vi "Module (Top Level).vi"(8 "error in":errorcluster) -> (0 "error out":errorcluster)   [LabVIEW 2017, in "myPAM.lvlib"]
uses:
  myPAM.lvlib
  Controls/RT Host - assistance definition.ctl
  Controls/RT Host - assistance options.ctl
  Controls/RT Host - form of control.ctl
  Controls/hCAAR - speed profile.ctl
  Controls/RT Host - assistance settings.ctl
  User Events/TypeDefs/Shutdown UE FGV Command.ctl
  Global TypeDefs/Registered Modules.ctl
  Public TypeDefs/Messages.ctl
  Public TypeDefs/Data for Logging.ctl
  <vilib>/Platform/TimedLoop/XDataNode/timing_clust.ctl
  <vilib>/Platform/TimedLoop/XDataNode/nitl_modes.ctl
  <vilib>/Platform/TimedLoop/XDataNode/wakeup.ctl
  Libraries/Real time filter/TypeDefs/Modes.ctl
  Public TypeDefs/Current Position Data.ctl
  <vilib>/FPGAPlugInAG/myRIO-1900/niLvFpga_Open_myRIO-1900.vi
  <vilib>/Utility/error.llb/Error Cluster From Error Code.vi
  <vilib>/rvi/errors/niLvFpgaAdjustHostInterfaceError.vi
  <vilib>/FPGAPlugInAG/myRIO-1900/niLvFpga_Run_myRIO-1900.vi
  <vilib>/FPGAPlugInAG/myRIO-1900/niLvFpga_Close_myRIO-1900.vi
  <vilib>/rvi/interface/nirviOpenFPGA/nirviOpenFPGA.xnode
  <instrlib>/Devantech SRF02/FPGA Example/Serial/Private/FPGA Reference.ctl
  FPGA Bitfiles/myPAM_FPGATarget_FPGA(TopLevel)_Z9iTYCZN6aI.lvbitx
  FPGA/FPGA (Top Level).vi
  <vilib>/rvi/interface/nirviReadWriteControl/nirviReadWriteControl.xnode
  <vilib>/rvi/interface/nirviMethod/nirviMethod.xnode
  <vilib>/Platform/TimedLoop/XDataNode/XDataNode.xnode
  <vilib>/rvi/interface/nirviCloseFPGA/nirviCloseFPGA.xnode
  Logger/Logger.lvlib
  Error Handler/Error Handler.lvlib
  Game/Game.lvlib
  <vilib>/Platform/TimedLoop/XDataNode/XDNodeRunTimeDep.lvlib
  WinHost/WinHost.lvlib
  Libraries/Real time filter/RealTimeFilter.lvlib
  NiFpgaLv.dll
panel:
  in  "g2":dbl=400.0 format="%#_13g"
  in  "g1":dbl=7100.0 format="%#_13g"
  in  "Parameters":T1={"Spring Stiffness"=9.0, "Deadzone Radius"=0.1, "Damping "=0.09}
  in  "Assistance Definition":T2={"Assistance Options"={"Assist Towards Target?"=TRUE, "Assist Ratchet?"=FALSE, "Form of Control?"=enum."Gen II", "Which Speed Profile?"=enum."Forward Skew"}, "Assistance Settings"={"Max Valley Width (mm)"=30.0, "Valley Width @ Tn (0-0.5)"=0.5, "Valley Width @ Tn-1 (0.5-1)"=0.5, "Valley Depth (0-1)"=1.0, "Stiffness (0-1)"=0.5, "Max Step Increment (mm)"=3.0, "Speed (0-1)"=0.33}}
  in  "Elbow":T7={"Spring Stiffness"=5.0, "Deadzone Radius"=0.01}
  in  "Shoulder":T7={"Spring Stiffness"=4.4, "Deadzone Radius"=0.01}
  out "LINK1_DEMAND":dbl
  out "LINK2_DEMAND":dbl
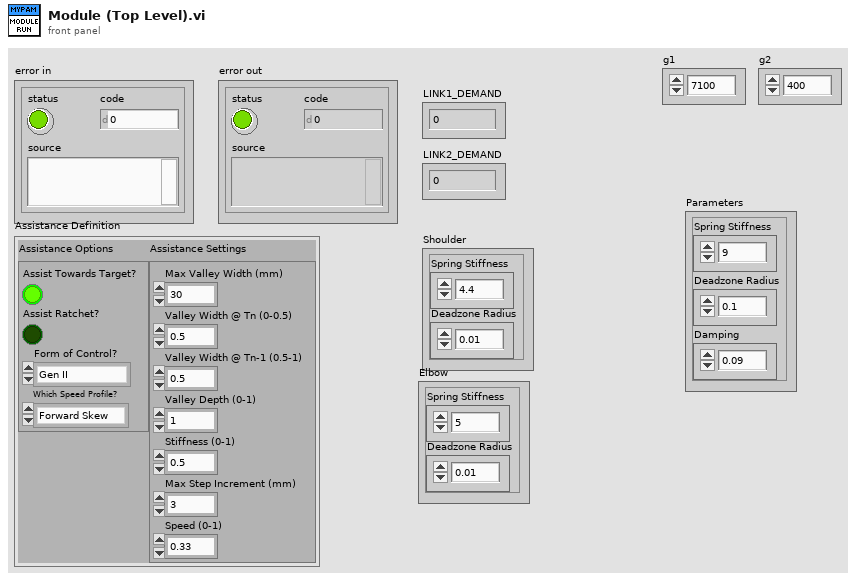
[diagram p1: front panel]
types:
  T1 = cluster{"Spring Stiffness":dbl, "Deadzone Radius":dbl, "Damping ":dbl}
  T2 = typedef "RT Host - assistance definition.ctl" = cluster{"Assistance Options":T3, "Assistance Settings":T6}
  T3 = typedef "RT Host - assistance options.ctl" = cluster{"Assist Towards Target?":bool, "Assist Ratchet?":bool, "Form of Control?":T4, "Which Speed Profile?":T5}
  T4 = typedef "RT Host - form of control.ctl" = enum16{"Baseline", "Gen II", "No Assist"}
  T5 = typedef "hCAAR - speed profile.ctl" = enum16{"Sine", "Sine With Initial Shunt", "Triangle", "Square", "Sawtooth", "Forward Skew", "User Defined"}
  T6 = typedef "RT Host - assistance settings.ctl" = cluster{"Max Valley Width (mm)":dbl, "Valley Width @ Tn (0-0.5)":dbl, "Valley Width @ Tn-1 (0.5-1)":dbl, "Valley Depth (0-1)":dbl, "Stiffness (0-1)":dbl, "Max Step Increment (mm)":dbl, "Speed (0-1)":dbl}
  T7 = cluster{"Spring Stiffness":dbl, "Deadzone Radius":dbl}
  T8 = typedef "Registered Modules.ctl" = enum16{"Controller", "DAQ", "Error Handler", "Game", "myPAM", "WinHost", "Logger"}
  T9 = typedef "Shutdown UE FGV Command.ctl" = enum16{"create", "get", "destroy"}
  T10 = typedef "WinHost.lvlib/Module Reference.ctl" = cluster{"calling module":T8, "module queues":T11, "module notifiers":T12}
  T11 = typedef "WinHost.lvlib/Module Queues.ctl" = cluster{"message queue":refnum<queue>, "STM queue":refnum<queue>}
  T12 = typedef "WinHost.lvlib/Module Notifiers.ctl" = cluster{"dummy notifier":refnum<notifier>}
  T13 = typedef "Game.lvlib/Module Reference.ctl" = cluster{"calling module":T8, "module queues":T14, "module notifiers":T15}
  T14 = typedef "Game.lvlib/Module Queues.ctl" = cluster{"message queue":refnum<queue>}
  T15 = typedef "Game.lvlib/Module Notifiers.ctl" = cluster{"dummy notifier":refnum<notifier>}
  T16 = typedef "Logger.lvlib/Module Reference.ctl" = cluster{"calling module":T8, "module queues":T17, "module notifiers":T18}
  T17 = typedef "Logger.lvlib/Module Queues.ctl" = cluster{"message queue":refnum<queue>}
  T18 = typedef "Logger.lvlib/Module Notifiers.ctl" = cluster{"dummy notifier":refnum<notifier>}
  T19 = typedef "myPAM.lvlib/Module Reference.ctl" = cluster{"calling module":T8, "module queues":T20, "module notifiers":T21}
  T20 = typedef "myPAM.lvlib/Module Queues.ctl" = cluster{"message queue":refnum<queue>}
  T21 = typedef "myPAM.lvlib/Module Notifiers.ctl" = cluster{"end eff. pos.":refnum<notifier>}
  T22 = typedef "Error Handler.lvlib/Module Reference.ctl" = cluster{"calling module":T8, "module queues":T23, "module notifiers":T24}
  T23 = typedef "Error Handler.lvlib/Module Queues.ctl" = cluster{"message queue":refnum<queue>}
  T24 = typedef "Error Handler.lvlib/Module Notifiers.ctl" = cluster{"dummy notifier":refnum<notifier>}
  T25 = cluster{"read mode":enum16{"polling", "blocking"}, "write mode":enum16{"polling", "blocking"}}
  T26 = typedef "myPAM.lvlib/Current Position Data.ctl" = cluster{"link 2 x (mm)":dbl, "link 2 y (mm)":dbl, "link 1 x (mm)":dbl, "link 1 y (mm)":dbl}
  T27 = typedef "XDNodeRunTimeDep.lvlib/timing_clust.ctl" = cluster{"Expected End [f-1]":u64, "Actual End [f-1]":u64, "Finished Late? [f-1]":bool, "Expected End [i-1]":u64, "Actual End [i-1]":u64, "Finished Late? [i-1]":bool, "Expected Start [i]":u64, "Actual Start [i]":u64, "Expected Start [f]":u64, "Actual Start [f]":u64, "Source Name":string, "Structure Name":string, "Period":i64, "Deadline":i64, "Offset":i64, "Start":i64, "Priority":i32, "Timeout":i32, "Mode":T28, "Wakeup Reason":T29, "Error":errorcluster, "Source Type":string, "Secondary Source Type":string, "Global End Time":u64, "Global Start Time":u64, "Frame Duration":u64, "Iteration Duration":u64, "Assigned CPU":i32, "I/O Scan Engine Mode":u32}
  T28 = typedef "XDNodeRunTimeDep.lvlib/nitl_modes.ctl" = enum32{"No Change", "Process missed periods, maintain original phase", "Discard missed periods, maintain original phase", "Process missed periods, ignore original phase", "Discard missed periods, ignore original phase"}
  T29 = typedef "XDNodeRunTimeDep.lvlib/wakeup.ctl" = enum32{"Normal", "Aborted", "Asynchronous wakeup", "Timing source error", "Timed loop error", "Timeout"}
  T30 = typedef "FPGA Reference.ctl" = refnum<k20>
  T31 = typedef "myPAM.lvlib/Messages.ctl" = enum16{"calibrate encoders", "enable motors", "disable motors", "operate", "shutdown"}
  T32 = typedef "myPAM.lvlib/Data for Logging.ctl" = cluster{"end effector x (mm)":dbl, "end effector y (mm)":dbl, "target x (mm)":dbl, "target y (mm)":dbl, "Theta 1":dbl, "Theta 2":dbl, "Omega 1":dbl, "Omega 2":dbl, "timestamp":dbl}
  T33 = typedef "myPAM.lvlib/RealTimeFilter.lvlib/Parameters.ctl" = cluster{"number of elements":i32, "start value":dbl, "sinusoidal profile":dbl[], "gaussian profile":dbl[]}
  T34 = typedef "myPAM.lvlib/RealTimeFilter.lvlib/Modes.ctl" = enum16{"Sinusoidal", "Gaussian"}
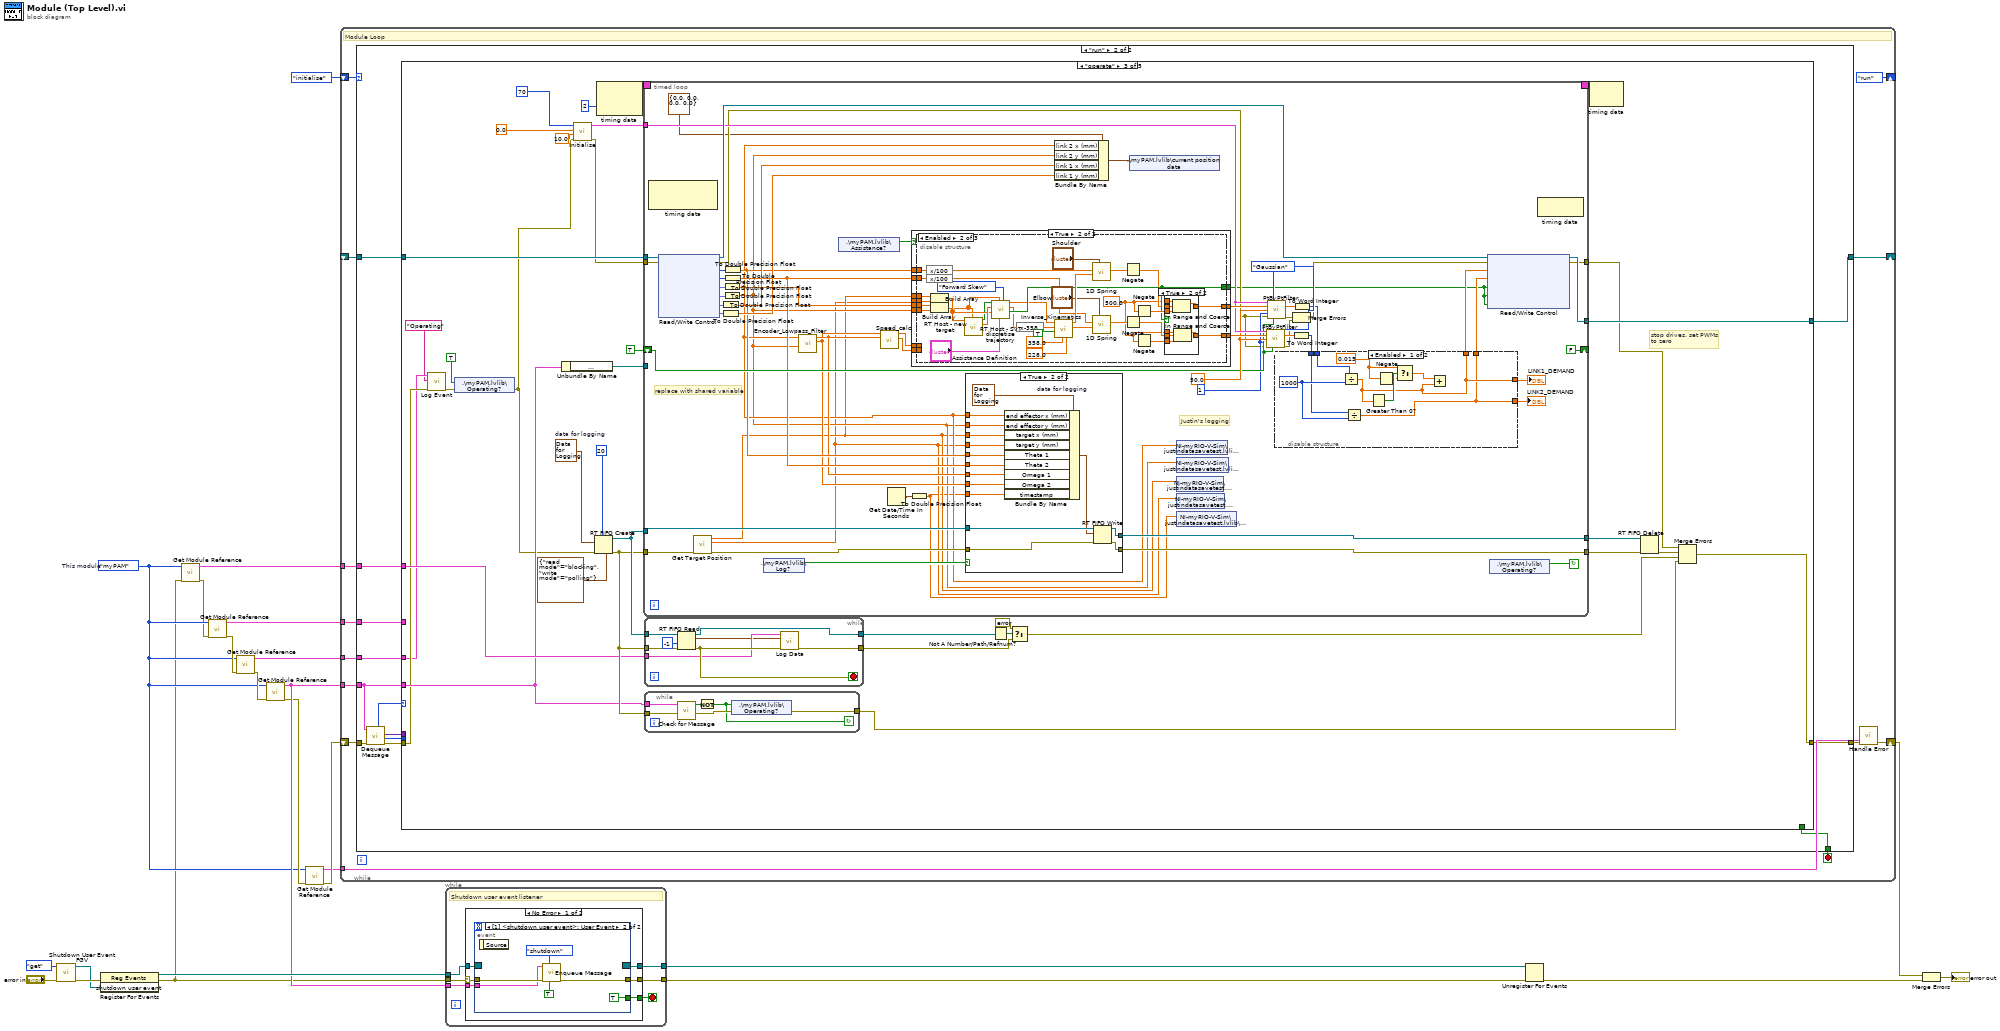
[diagram p0: block diagram]
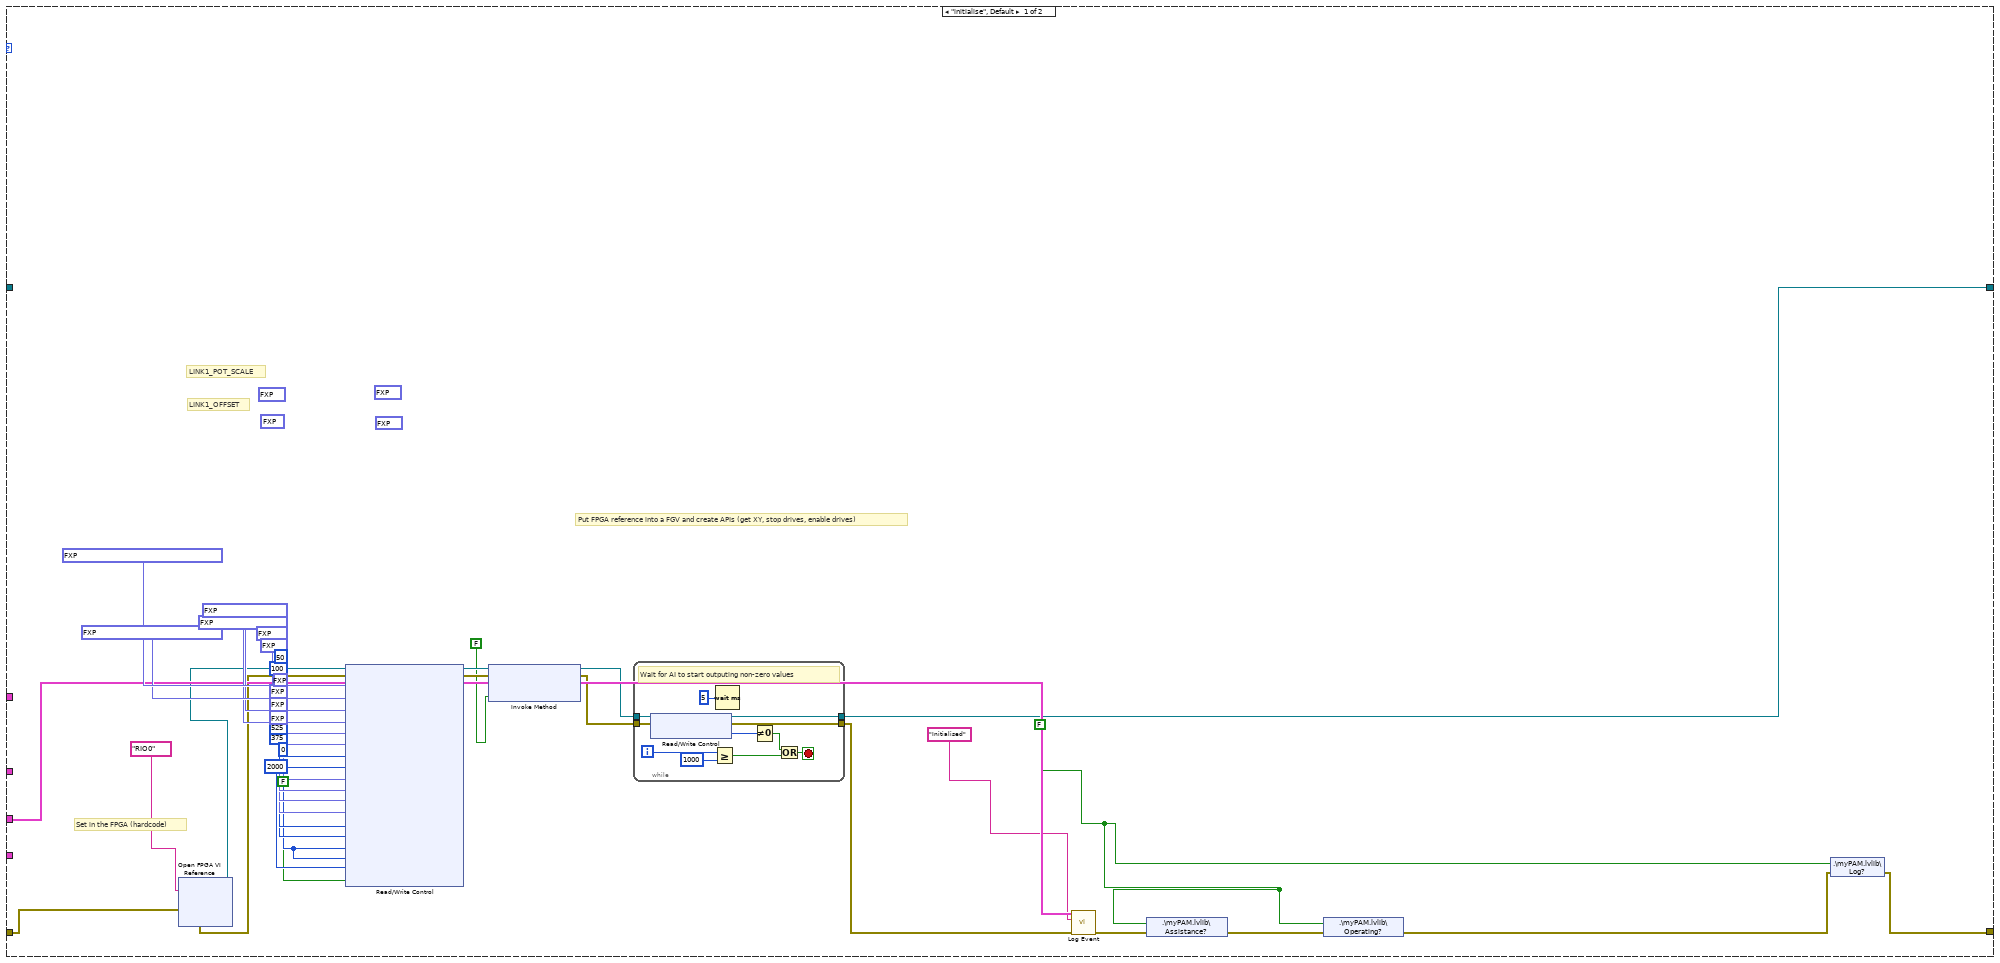
[diagram p2: hidden frame]
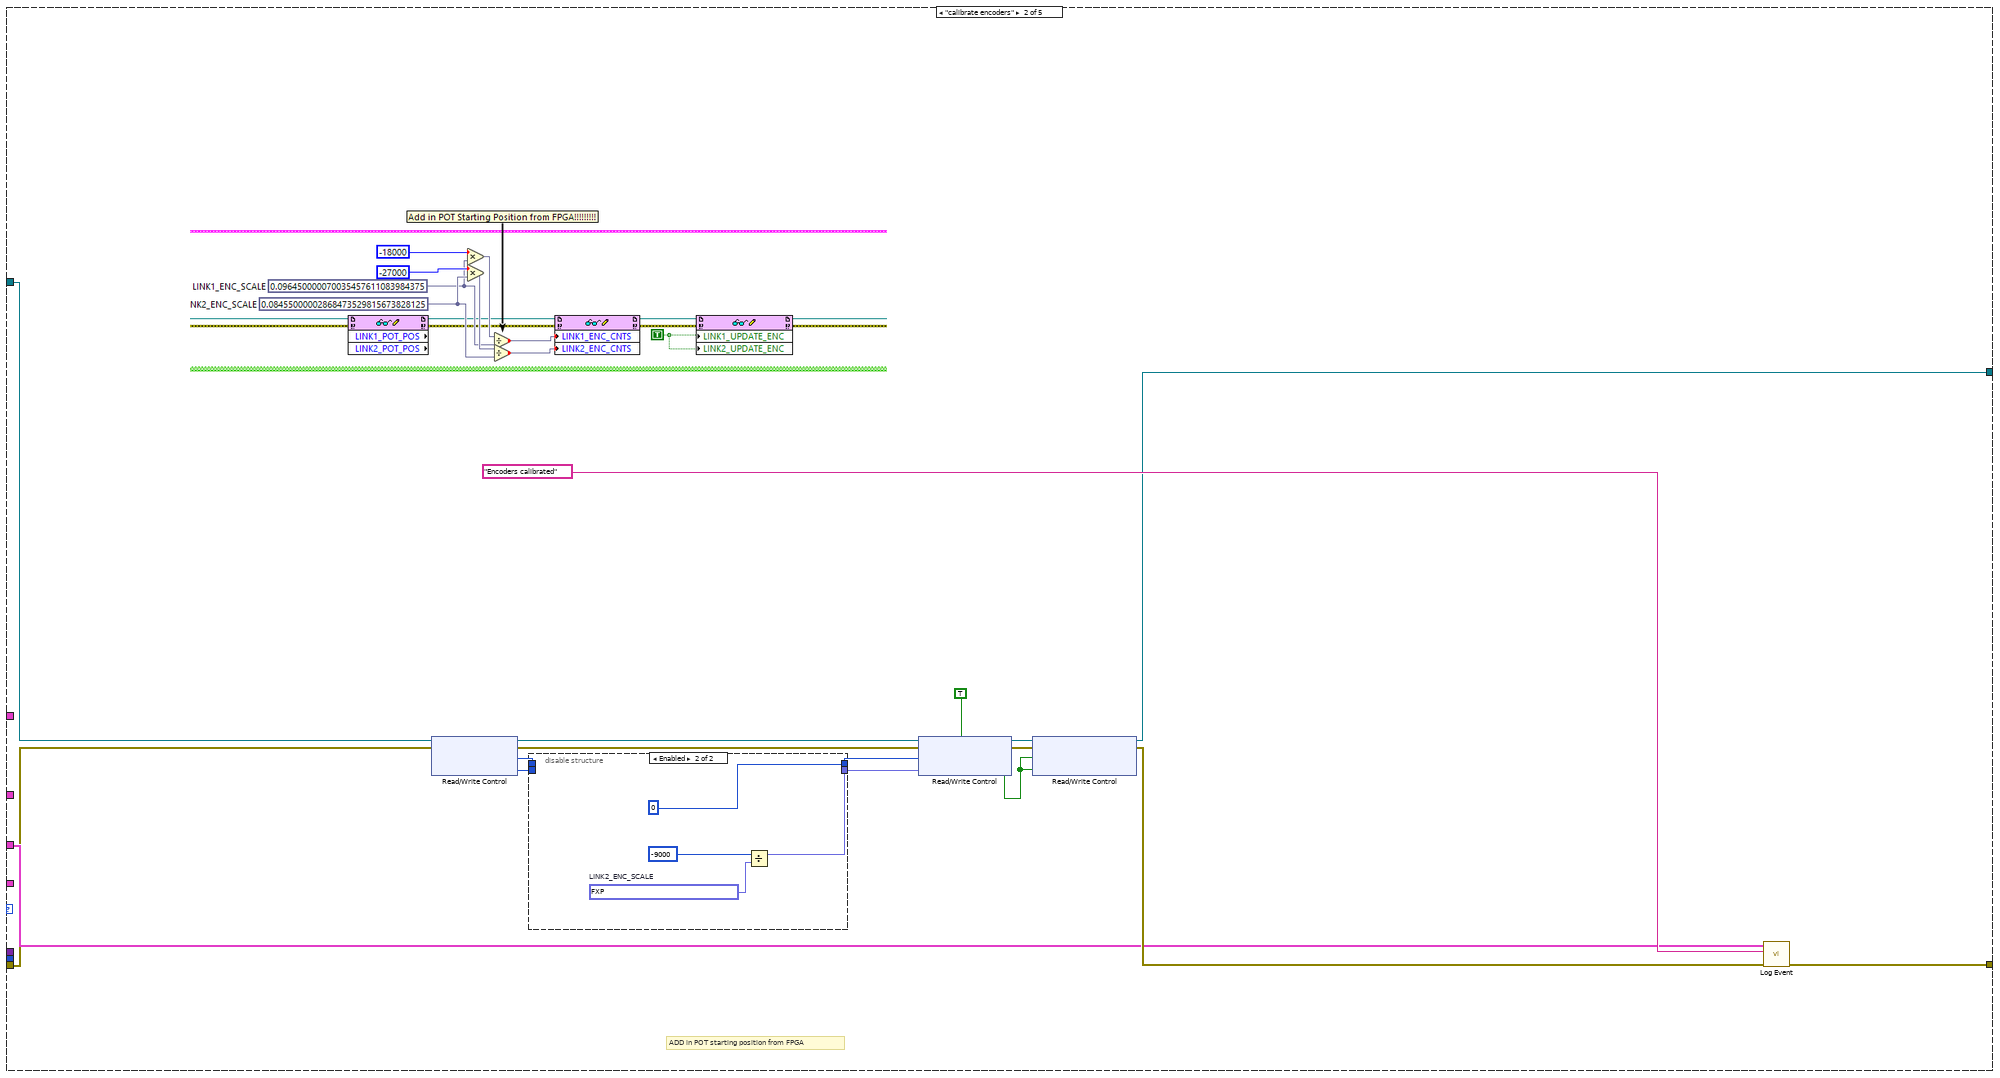
[diagram p4: hidden frame]
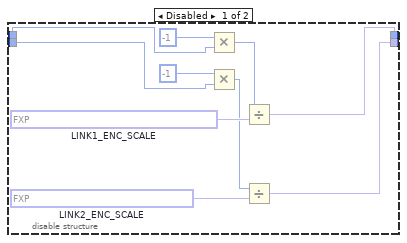
[diagram p5: hidden frame]
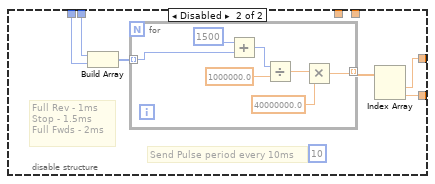
[diagram p6: hidden frame]
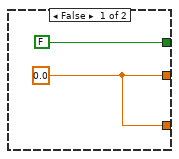
[diagram p7: hidden frame]
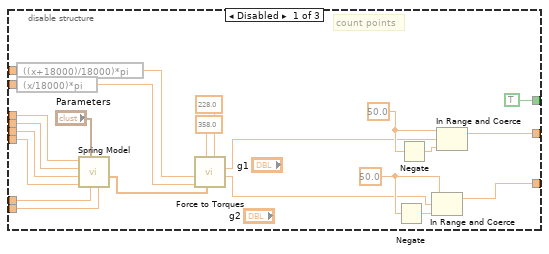
[diagram p8: hidden frame]
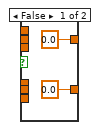
[diagram p9: hidden frame]
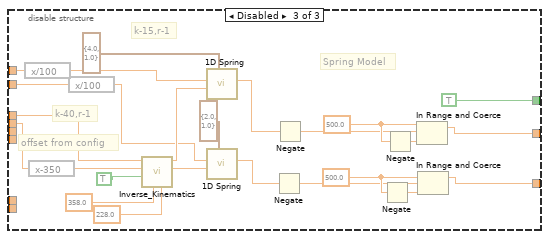
[diagram p10: hidden frame]
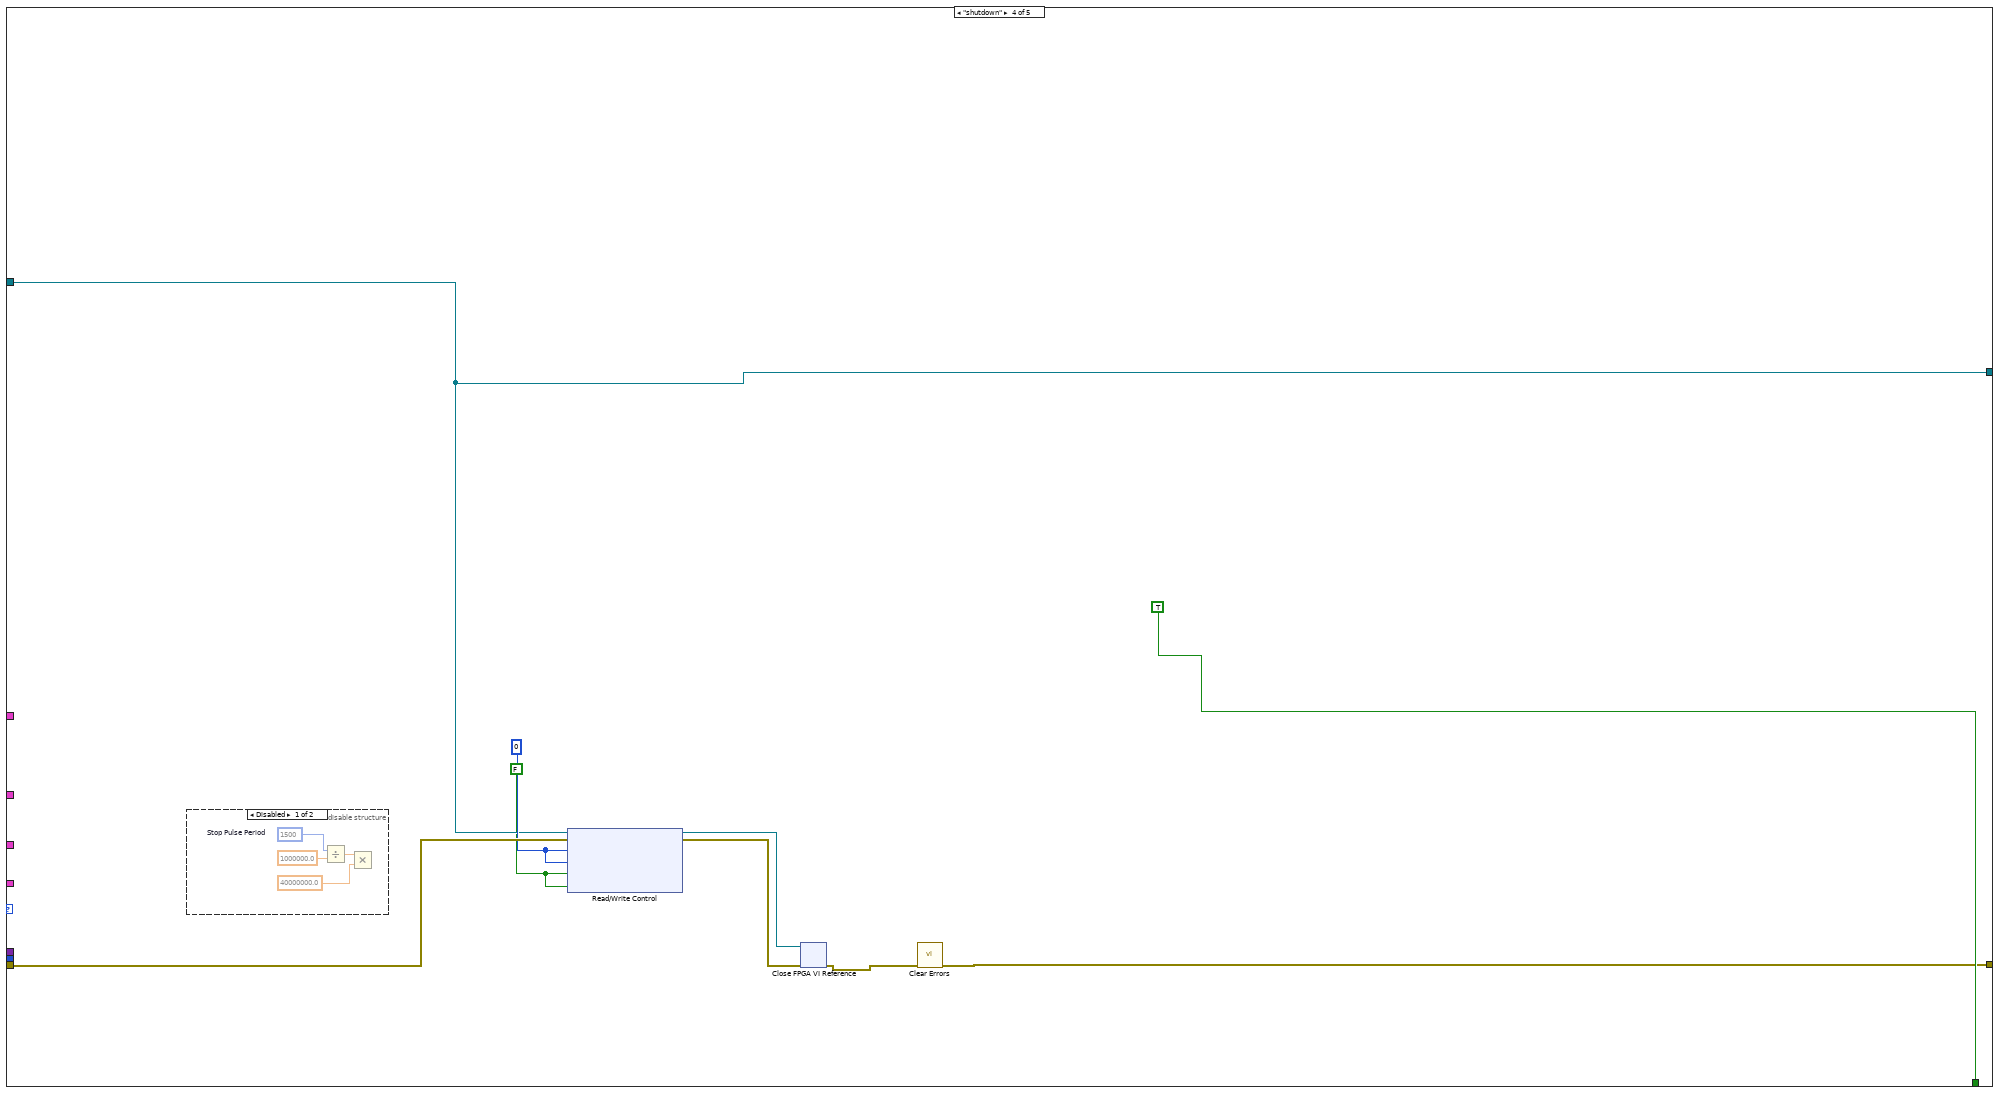
[diagram p12: hidden frame]
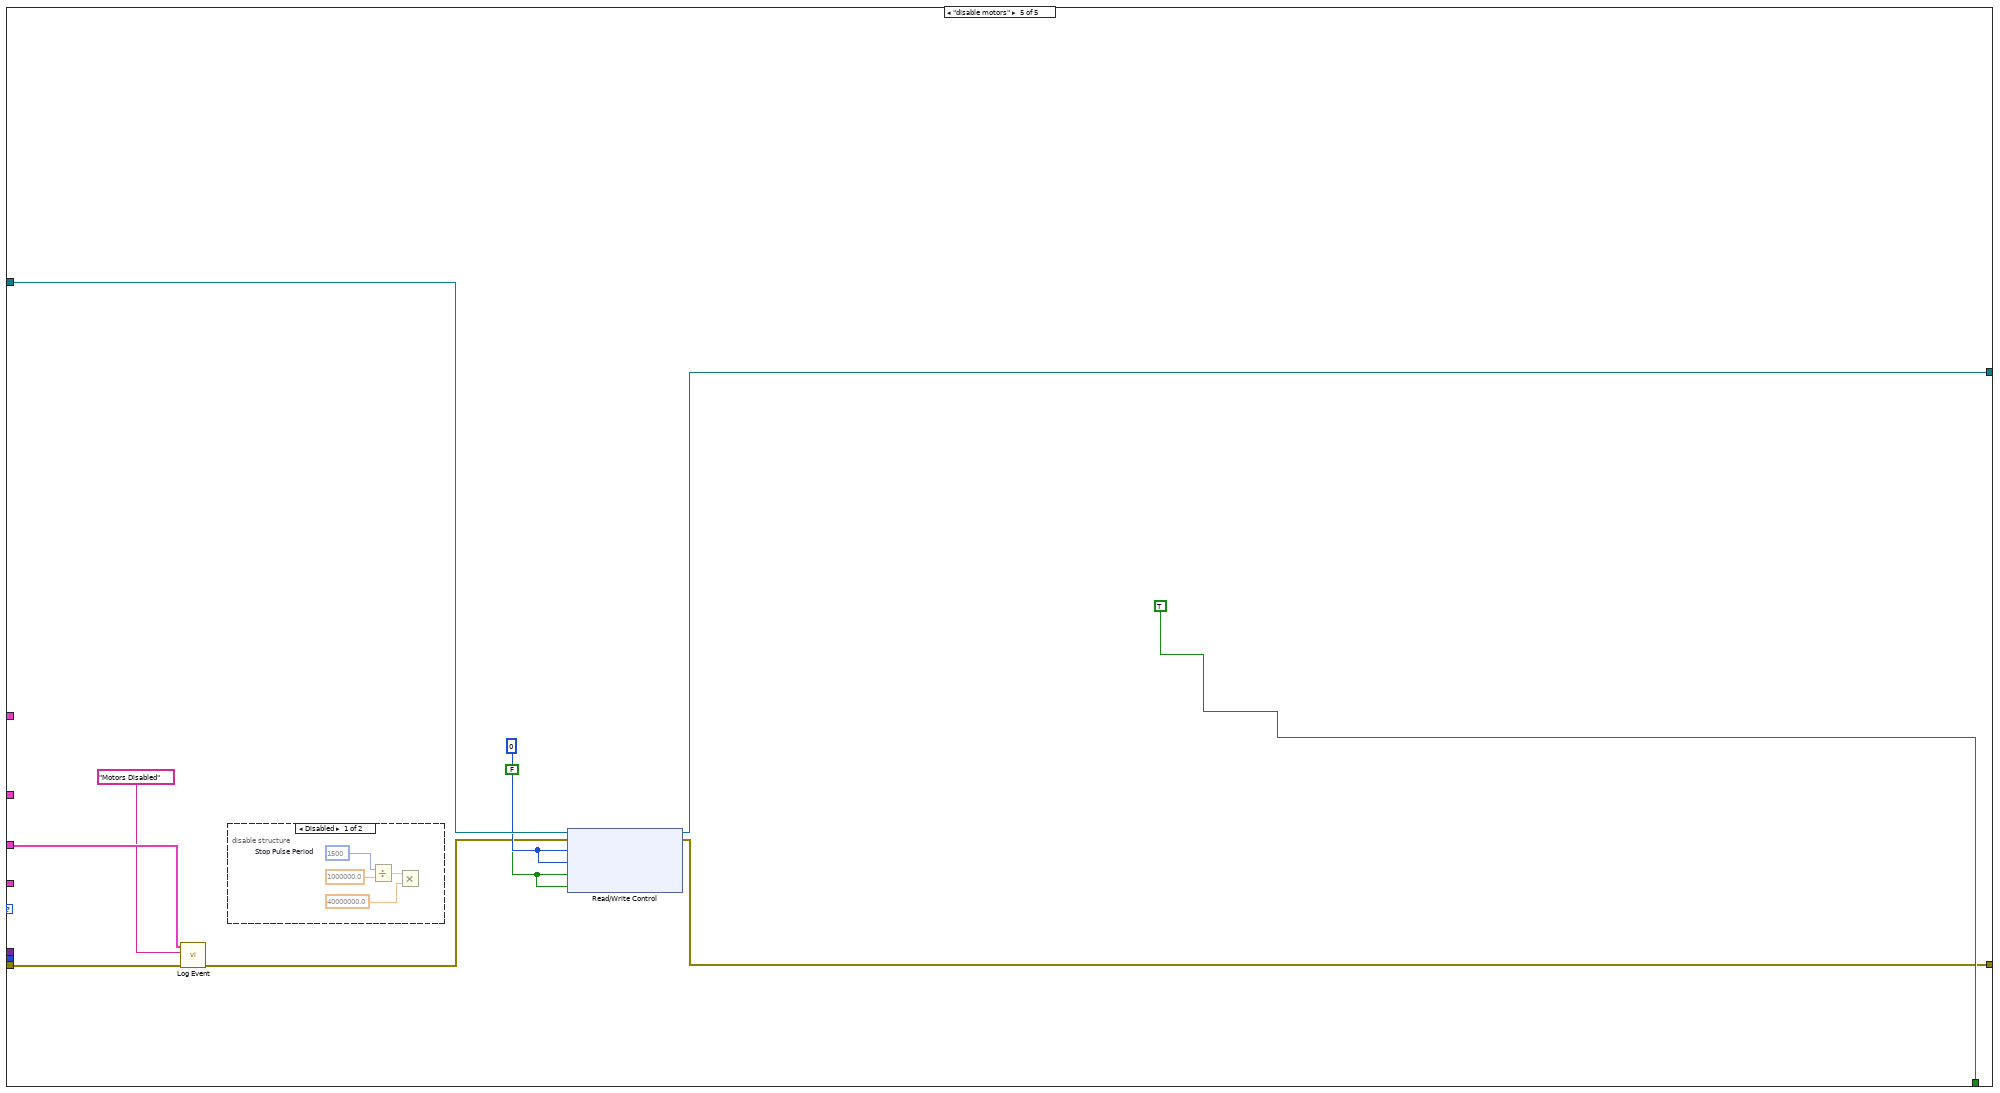
[diagram p14: hidden frame]
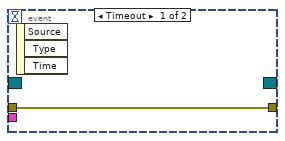
[diagram p16: hidden frame]
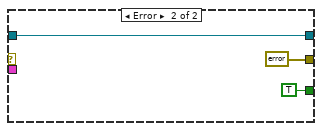
[diagram p17: hidden frame]
diagram:
  w4 = Registered_Modules."myPAM"  # This module
  n1 = call "Shutdown User Event FGV.vi"("error in"="error in", "command"=Shutdown_UE_FGV_Command."get" ("Command")) -> ("error out"=w18:errorcluster, "shutdown user event"=w17:refnum<user-event>)  [unwired: 8 in]
  n2 = register-events(error in=w18, w17) -> (reference out=w22:refnum<event-registration>, error out=w3:errorcluster)  [unwired: 1 in]
  n3 = call "Get Module Reference.vi"("error in"=w3, "calling module"=w4) -> ("error out"=w2:errorcluster, "module reference"=w1:T10)  [unwired: 8 in]
  n4 = call "Get Module Reference.vi"("error in"=w2, "calling module"=w4) -> ("error out"=w8:errorcluster, "module reference"=w5:T13)  [unwired: 8 in]
  n5 = call "Get Module Reference.vi"("error in"=w8, "calling module"=w4) -> ("error out"=w7:errorcluster, "module reference"=w6:T16)  [unwired: 8 in]
  n6 = call "Get Module Reference.vi"("error in"=w7, "calling module"=w4) -> ("error out"=w11:errorcluster, "module reference"=w13:T19)  [unwired: 8 in]
  n7 = call "Get Module Reference.vi"("error in"=w11, "calling module"=w4) -> ("error out"=w10:errorcluster, "module reference"=w9:T22)  [unwired: 8 in]
  n8 = while {
    shift-right: [w29] -> w20
    shift-left: w10 -> [w32]
    tunnel: w13 -> [w36]
    shift-right: [w24] -> _
    shift-left: _ -> [w35]
    shift-right: [enum16{"initialise", "run"}."run"] -> _
    shift-left: enum16{"initialise", "run"}."initialise" -> [w34]
    tunnel: w9 -> [w28]
    tunnel: w6 -> [w27]
    tunnel: w5 -> [w26]
    tunnel: w1 -> [w25]
    stop <- w31 stop-if-true
    # "Module Loop"
    n9 = case shown="\"run\"" w34 {
      tunnel: [w42 w95] -> w30
      tunnel: w36 -> [_ w85]
      tunnel: w35 -> [_ w90]
      tunnel: w32 -> [w57 w88]
      tunnel: [_ w89] -> w31
      tunnel: w27 -> [w63 w87]
      tunnel: w26 -> [_ w86]
      tunnel: w25 -> [_ w84]
      tunnel: [w45 w83] -> w24
      frame "initialise", Default {
        (unwired) fxp<+/-,16,16> 15788.0 ("LINK2_OFFSET")
        (unwired) fxp<+/-,32,16> -3352.0 ("LINK2_POT_SCALE")
        (unwired) fxp<+/-,16,16> 5308.0 ("LINK1_OFFSET")
        (unwired) fxp<+/-,32,16> -3396.0 ("LINK1_POT_SCALE")
        w39 = i16 0
        w41 = FALSE ("Enabled?")
        # "LINK1_OFFSET"
        # "LINK1_POT_SCALE"
        # "Set in the FPGA (hardcode)"
        # "Put FPGA reference into a FGV and create APIs (get XY, stop drives, enable drives)"
        n10 = xnode "Open FPGA VI Reference"("error in"=w57, "resource name"=tag "RIO0") -> ("FPGA VI Reference Out"=w56:T30, "error out"=w62:errorcluster)
        n11 = xnode "Read/Write Control"("FPGA VI Reference In"=w56, "error in"=w62, "LINK1_ENC_SCALE"=fxp<+,32,0> 0.21972699998877943, "LINK2_ENC_SCALE"=fxp<+,32,0> 0.12555800005793571, "LINK1_POT_SCALE"=fxp<+/-,32,16> 8.229995727539062, "LINK2_POT_SCALE"=fxp<+/-,32,16> -4.1016998291015625, "LINK1_OFFSET"=fxp<+/-,16,16> -11376.0, "LINK2_OFFSET"=fxp<+/-,16,16> 13125.0, "ENC_DEBOUNCE_CYCLES"=u16 50, "AI_POT_LOOP_US"=u16 100, "X_OFFSET_MM"=fxp<+/-,33,15> 0.0, "Y_OFFSET_MM"=fxp<+/-,33,15> 358.0, "LINK1_LENGTH_MM"=fxp<+,16,12> 358.0, "LINK2_LENGTH_MM"=fxp<+,16,12> 228.0, "LINK1_PWM_MAX"=i16 525, "LINK2_PWM_MAX"=i16 375 ("LINK1_PWM_MAX"), "LINK1_DEMAND_PWM"=w39, "LINK2_DEMAND_PWM"=w39, "PWM Period Loops"=2000, "Enable Output V"=FALSE) -> ("FPGA VI Reference Out"=w50:T30, "error out"=w51:errorcluster)
        n12 = xnode "Invoke Method"("FPGA VI Reference In"=w50, "error in"=w51, "Wait Until Done (F)"=FALSE) -> ("FPGA VI Reference Out"=w49:T30, "error out"=w48:errorcluster)
        n13 = while {
          tunnel: w49 -> [w82]
          tunnel: w48 -> [w74]
          tunnel: [w73] -> w45
          tunnel: [w72] -> w47
          i -> [w78]
          stop <- w80 stop-if-true
          # "Wait for AI to start outputing non-zero values"
          n14 = xnode "Read/Write Control"("FPGA VI Reference In"=w82, "error in"=w74) -> ("FPGA VI Reference Out"=w73:T30, "error out"=w72:errorcluster, "LINK1_POT_POS"=w81:i32)
          n15 = Greater Or Equal?(x=w78, y=1000) -> (x >= y?=w75:bool)
          n16 = Wait (ms)(milliseconds to wait=u32 5) -> ()  [unwired: 1 out]
          n17 = Not Equal To 0?(x=w81) -> (x != 0?=w79:bool)
          n18 = Or(x=w79, y=w75) -> (x .or. y?=w80:bool)
        }
        n19 = call "Log Event.vi"("error in"=w47, "event"="Initialised" ("string"), "module reference in"=w63) -> ("error out"=w53:errorcluster)  [unwired: 7 in, 1 out]
        n20 = shared-variable ".\\myPAM.lvlib\\Assistance?"(w41, error in=w53) -> (error out=w40:errorcluster)
        n21 = shared-variable ".\\myPAM.lvlib\\Operating?"(w41, error in=w40) -> (error out=w43:errorcluster)
        n22 = shared-variable ".\\myPAM.lvlib\\Log?"(w41, error in=w43) -> (error out=w42:errorcluster)
      }
      frame "run" {
        n23 = call "Dequeue Message.vi"("error in"=w88, "module reference in"=w85) -> ("error out"=w93:errorcluster, "source"=w91:T8, "data"=w92:variant, "message"=w94:T31)  [unwired: 5 in, 1 out]
        n24 = case shown="\"operate\"" w94 {
          tunnel: [w97 w102 w144 w390 w405] -> w95
          tunnel: w93 -> [w97 w100 w140 w388 w401]
          tunnel: w92 -> [_ _ _ _ _]
          tunnel: w91 -> [_ _ _ _ _]
          tunnel: w90 -> [w96 w106 w160 w385 w404]
          tunnel: [_ _ _ TRUE TRUE] -> w89
          tunnel: w87 -> [_ w103 w139 _ w399]
          tunnel: w86 -> [_ _ _ _ _]
          tunnel: w85 -> [_ _ w142 _ _]
          tunnel: [w96 w101 w153 w385 w402] -> w83
          tunnel: w84 -> [_ _ w143 _ _]
          frame Default {
          }
          frame "calibrate encoders" {
            w107 = TRUE
            # "ADD in POT starting position from FPGA"
            n25 = xnode "Read/Write Control"("FPGA VI Reference In"=w106, "error in"=w100) -> ("FPGA VI Reference Out"=w110:T30, "error out"=w111:errorcluster, "LINK1_POT_POS"=w99:i32, "LINK2_POT_POS"=w98:i32)
            n26 = disable-structure shown="Enabled" {
              disable-tunnel: [w123 0] -> w113
              disable-tunnel: [w122 w125] -> w112
              disable-tunnel: w99 -> [w115 _]
              disable-tunnel: w98 -> [w114 _]
              frame Disabled {
                w118 = fxp<+,32,0> 0.12555800005793571  # LINK2_ENC_SCALE
                w119 = fxp<+/-,32,0> 0.21972699998877943  # LINK1_ENC_SCALE
                n27 = Multiply(x=-1, y=w115) -> (x*y=w117:i32)
                n28 = Multiply(x=-1, y=w114) -> (x*y=w116:i32)
                n29 = Divide(x=w117, y=w119) -> (x/y=w123:fxp<+/-,64,65>)
                n30 = Divide(x=w116, y=w118) -> (x/y=w122:fxp<+/-,64,64>)
              }
              frame Enabled {
                w124 = fxp<+,32,0> 0.12555800005793571  # LINK2_ENC_SCALE
                n31 = Divide(x=-9000, y=w124) -> (x/y=w125:fxp<+/-,64,64>)
              }
            }
            n32 = xnode "Read/Write Control"("FPGA VI Reference In"=w110, "error in"=w111, "LINK1_ENC_CNTS"=w113, "LINK2_ENC_CNTS"=w112) -> ("FPGA VI Reference Out"=w109:T30, "error out"=w108:errorcluster)
            n33 = xnode "Read/Write Control"("FPGA VI Reference In"=w109, "error in"=w108, "LINK1_UPDATE_ENC"=w107, "LINK2_UPDATE_ENC"=w107) -> ("FPGA VI Reference Out"=w101:T30, "error out"=w105:errorcluster)
            n34 = call "Log Event.vi"("error in"=w105, "event"="Encoders calibrated", "module reference in"=w103) -> ("error out"=w102:errorcluster)  [unwired: 7 in, 1 out]
          }
          frame "operate" {
            w157 = T32 {"end effector x (mm)"=0.0, "end effector y (mm)"=0.0, "target x (mm)"=0.0, "target y (mm)"=0.0, "Theta 1"=0.0, "Theta 2"=0.0, "Omega 1"=0.0, "Omega 2"=0.0, "timestamp"=0.0}  # data for logging
            # "stop drives, set PWMs\nto zero"
            n35 = call "Log Event.vi"("error in"=w140, "event"="Operating", "module reference in"=w139) -> ("error out"=w137:errorcluster)  [unwired: 7 in, 1 out]
            n36 = shared-variable ".\\myPAM.lvlib\\Operating?"(TRUE ("Operating?"), error in=w137) -> (error out=w130:errorcluster)
            n37 = Unbundle By Name(w142) -> ("module notifiers.end eff. pos."=w161:refnum<notifier>)
            n38 = call "Initialise.vi"("error in (no error)"=w130, "gaussian stdev (elements)"=10.0, "start value"=0.0, "number of elements (max 2048)"=70) -> ("error out"=w129:errorcluster, "parameter cluster"=w135:T33)  [unwired: 6 in]
            n39 = RT FIFO Create(1:w157, 3:w130, 4:u32 20 ("size (10)"), 7:T25 {"read mode"=enum."blocking", "write mode"=enum."polling"} ("r/w modes (polling,polling)")) -> (8:w154:refnum<k33>, 11:w148:errorcluster)  [unwired: 4 in, 1 out]
            n40 = node-c288(i64 2 ("Period")) -> (w163:T27)  [unwired: 1 in]
            n41 = timed-loop {
              timing: w163 -> [_]
              timing-out: [_] -> w162
              tunnel: w160 -> [w218]
              tunnel: w161 -> [_]
              tunnel: w148 -> [w185]
              tunnel: w154 -> [w216]
              tunnel: [w215] -> w156
              tunnel: [w214] -> w155
              tunnel: [w208] -> w153
              tunnel: w129 -> [w213]
              tunnel: w135 -> [w202]
              shift-right: [FALSE] -> _
              shift-left: TRUE -> [w198]
              tunnel: [w192] -> w128
              stop <- w219 continue-if-true
              w197 = i64 1 ("dt")
              w201 = 50.0 ("max speed")
              w199 = Modes."Gaussian" ("Mode")
              # "Justin's logging"
              # "replace with shared variable"
              n42 = node-c288() -> ()  [unwired: 1 in, 2 out]
              n43 = xnode "Read/Write Control"("FPGA VI Reference In"=w218, "error in"=w213) -> ("FPGA VI Reference Out"=w207:T30, "error out"=w196:errorcluster, "LINK1_ENC_POS"=w210:i32, "LINK2_ENC_POS"=w209:i32, "LINK2_X_MM"=w212:fxp<+/-,34,16>, "LINK2_Y_MM"=w211:fxp<+/-,34,16>, "LINK1_X_MM"=w189:fxp<+/-,34,16>, "LINK1_Y_MM"=w188:fxp<+/-,34,16>)
              n44 = call "Get Target Position.vi"("error in"=w185) -> ("error out"=w184:errorcluster, "target y (mm)"=w165:dbl, "target x (mm)"=w166:dbl)  [unwired: 8 in]
              n45 = To Double Precision Float(number=w189) -> (double precision float=w187:dbl)
              n46 = To Double Precision Float(number=w188) -> (double precision float=w186:dbl)
              n47 = To Double Precision Float(number=w212) -> (double precision float=w168:dbl)
              n48 = To Double Precision Float(number=w211) -> (double precision float=w167:dbl)
              n49 = To Double Precision Float(number=w210) -> (double precision float=w172:dbl)
              n50 = To Double Precision Float(number=w209) -> (double precision float=w173:dbl)
              n51 = shared-variable ".\\myPAM.lvlib\\Log?"() -> (w217:bool)  [unwired: 1 in, 1 out]
              n52 = call "Encoder_Lowpass_Filter.vi"("LINK2_ENC_POS"=w167, "LINK1_ENC_POS"=w168) -> ("LINK2_ENC_POS_FILTERED"=w170:dbl, "LINK1_ENC_POS_FILTERED"=w171:dbl)  [unwired: 6 in]
              n53 = shared-variable ".\\myPAM.lvlib\\Assistance?"() -> (w183:bool)  [unwired: 1 in, 1 out]
              n54 = call "Speed_calc.vi"("X"=w171, "Y"=w170) -> ("Vy"=w174:dbl, "Vx"=w175:dbl)  [unwired: 8 in]
              n55 = Get Date/Time In Seconds() -> (seconds since 1Jan1904=w169:timestamp)
              n56 = To Double Precision Float(number=w169) -> (double precision float=w164:dbl)
              n57 = case shown="True" w183 {
                tunnel: w168 -> [_ w254]
                tunnel: w167 -> [_ w253]
                tunnel: w172 -> [_ w252]
                tunnel: w173 -> [_ w251]
                tunnel: w165 -> [_ w250]
                tunnel: w166 -> [_ w249]
                tunnel: [w243 w247] -> w206
                tunnel: [w243 w246] -> w204
                tunnel: [FALSE w248] -> w176
                tunnel: w175 -> [_ w245]
                tunnel: w174 -> [_ w244]
                frame False {
                  w243 = 0.0
                }
                frame True {
                  n58 = disable-structure shown="Enabled" {
                    disable-tunnel: w254 -> [w277 w295 _]
                    disable-tunnel: w253 -> [w276 w294 _]
                    disable-tunnel: w252 -> [w274 w302 w330]
                    disable-tunnel: w251 -> [w273 w300 w328]
                    disable-tunnel: w250 -> [w270 w297 w326]
                    disable-tunnel: w249 -> [w269 w296 w324]
                    disable-tunnel: [TRUE w289 TRUE] -> w248
                    disable-tunnel: [w263 w306 w339] -> w247
                    disable-tunnel: [w262 w305 w338] -> w246
                    disable-tunnel: w245 -> [w259 _ _]
                    disable-tunnel: w244 -> [w258 _ _]
                    frame Disabled {
                      w265 = 50.0 ("LINK1_PWM_MAX")
                      w267 = 50.0 ("LINK1_PWM_MAX")
                      # "count points"
                      n59 = expression code="((x+18000)/18000)*pi" ("degrees to radians")(w274) -> (w261:dbl)
                      n60 = expression code="(x/18000)*pi" ("degrees to radians")(w273) -> (w260:dbl)
                      n61 = call "Spring Model.vi"("Vy"=w258, "Vx"=w259, "Parameters"="Parameters", "Current Y"=w276, "Current X"=w277, "Target Y"=w270, "Target X"=w269) -> ("F_vector"=w257:cdb[])  [unwired: 4 in]
                      n62 = call "Force to Torques.vi"("L2"=228.0, "F_vector"=w257, "L1"=358.0, "th2"=w260, "th1"=w261) -> ("T2"=w255:dbl, "T1"=w256:dbl)  [unwired: 4 in]
                      n63 = Negate(x=w265) -> (-x=w266:dbl)
                      n64 = Negate(x=w267) -> (-x=w268:dbl)
                      n65 = In Range and Coerce(upper limit=w265, x=w255, lower limit=w266) -> (coerced(x)=w262:dbl)  [unwired: 1 out]
                      n66 = In Range and Coerce(upper limit=w267, x=w256, lower limit=w268) -> (coerced(x)=w263:dbl)  [unwired: 1 out]
                    }
                    frame Enabled {
                      w278 = 500.0 ("LINK1_PWM_MAX")
                      n67 = expression code="x/100" ("degrees to radians")(w302) -> (w301:dbl)
                      n68 = expression code="x/100" ("degrees to radians")(w300) -> (w299:dbl)
                      n69 = Build Array(w296, w297) -> (w292:dbl[])
                      n70 = Build Array(w295, w294) -> (w291:dbl[])
                      n71 = call "RT Host - new target.vi"("Current Pos (mm)"=w291, "Target Pos (mm)"=w292) -> ("Previous Target Pos (mm)"=w293:dbl[], "New Target?"=w290:bool)  [unwired: 7 in, 1 out]
                      n72 = call "RT Host - SvT discretise trajectory.vi"("Which speed profile?"=hCAAR_-_speed_profile."Forward Skew", "Assistance Definition"="Assistance Definition", "Current Joy Global W/S Pos (mm)"=w291, "Target Global W/S Pos (mm)"=w292, "Previous Target Global W/S Pos (mm)"=w293, "New Target?"=w290) -> ("Speed Assistance?"=w289:bool, "Global Ydes (mm)"=w288:dbl, "Global Xdes (mm)"=w287:dbl)  [unwired: 1 in, 2 out]
                      n73 = expression code="x-358" ("degrees to radians")(w288) -> (w298:dbl)
                      n74 = call "Inverse_Kinematics.vi"("arm2 length (mm)"=228.0 ("L1"), "arm1 length (mm)"=358.0 ("L2"), "arm direction"=TRUE, "y (mm)"=w298, "x (mm)"=w287) -> ("th2"=w303:dbl, "th1"=w304:dbl)  [unwired: 5 in]
                      n75 = call "1D Spring.vi"("Parameters"="Shoulder", "desired pos"=w304, "current pos"=w301) -> ("output"=w282:dbl)  [unwired: 8 in]
                      n76 = call "1D Spring.vi"("Parameters"="Elbow", "desired pos"=w303, "current pos"=w299) -> ("output"=w281:dbl)  [unwired: 8 in]
                      n77 = Negate(x=w282) -> (-x=w280:dbl)
                      n78 = Negate(x=w281) -> (-x=w279:dbl)
                      n79 = Negate(x=w278) -> (-x=w308:dbl)
                      n80 = Negate(x=w278) -> (-x=w307:dbl)
                      n81 = case shown="True" w289 {
                        tunnel: w308 -> [_ w321]
                        tunnel: w278 -> [_ w320]
                        tunnel: w307 -> [_ w319]
                        tunnel: w278 -> [_ w318]
                        tunnel: [0.0 ("LINK1_PWM_MAX") w317] -> w306
                        tunnel: [0.0 ("LINK1_PWM_MAX") w316] -> w305
                        tunnel: w280 -> [_ w315]
                        tunnel: w279 -> [_ w314]
                        frame False {
                        }
                        frame True {
                          n82 = In Range and Coerce(upper limit=w320, x=w315, lower limit=w321) -> (coerced(x)=w317:dbl)  [unwired: 1 out]
                          n83 = In Range and Coerce(upper limit=w318, x=w314, lower limit=w319) -> (coerced(x)=w316:dbl)  [unwired: 1 out]
                        }
                      }
                    }
                    frame Disabled {
                      w340 = 500.0 ("LINK1_PWM_MAX")
                      w342 = 500.0 ("LINK1_PWM_MAX")
                      # "k-40,r-1"
                      # "k-15,r-1"
                      # "Spring Model"
                      # "offset from config"
                      n84 = expression code="x/100" ("degrees to radians")(w330) -> (w329:dbl)
                      n85 = expression code="x-350" ("degrees to radians")(w326) -> (w325:dbl)
                      n86 = expression code="x/100" ("degrees to radians")(w328) -> (w327:dbl)
                      n87 = call "Inverse_Kinematics.vi"("arm2 length (mm)"=228.0 ("L1"), "arm1 length (mm)"=358.0 ("L2"), "arm direction"=TRUE, "y (mm)"=w325, "x (mm)"=w324) -> ("th2"=w335:dbl, "th1"=w336:dbl)  [unwired: 5 in]
                      n88 = call "1D Spring.vi"("Parameters"=T7 {"Spring Stiffness"=4.0, "Deadzone Radius"=1.0}, "desired pos"=w336, "current pos"=w329) -> ("output"=w332:dbl)  [unwired: 8 in]
                      n89 = call "1D Spring.vi"("Parameters"=T7 {"Spring Stiffness"=2.0, "Deadzone Radius"=1.0} ("Parameters 2"), "desired pos"=w335, "current pos"=w327) -> ("output"=w333:dbl)  [unwired: 8 in]
                      n90 = Negate(x=w333) -> (-x=w322:dbl)
                      n91 = Negate(x=w332) -> (-x=w331:dbl)
                      n92 = Negate(x=w340) -> (-x=w341:dbl)
                      n93 = Negate(x=w342) -> (-x=w343:dbl)
                      n94 = In Range and Coerce(upper limit=w342, x=w331, lower limit=w343) -> (coerced(x)=w339:dbl)  [unwired: 1 out]
                      n95 = In Range and Coerce(upper limit=w340, x=w322, lower limit=w341) -> (coerced(x)=w338:dbl)  [unwired: 1 out]
                    }
                  }
                }
              }
              n96 = case shown="True" w217 {
                tunnel: w168 -> [_ w363]
                tunnel: w167 -> [_ w362]
                tunnel: w166 -> [_ w361]
                tunnel: w165 -> [_ w360]
                tunnel: w216 -> [w348 w358]
                tunnel: w184 -> [w347 w357]
                tunnel: [w348 w355] -> w215
                tunnel: [w347 w354] -> w214
                tunnel: w172 -> [_ w353]
                tunnel: w173 -> [_ w352]
                tunnel: w171 -> [_ w351]
                tunnel: w170 -> [_ w350]
                tunnel: w164 -> [_ w349]
                frame False {
                }
                frame True {
                  w359 = T32 {"end effector x (mm)"=0.0, "end effector y (mm)"=0.0, "target x (mm)"=0.0, "target y (mm)"=0.0, "Theta 1"=0.0, "Theta 2"=0.0, "Omega 1"=0.0, "Omega 2"=0.0, "timestamp"=0.0}  # data for logging
                  n97 = Bundle By Name(cluster=w359, "end effector x (mm)"=w363, "end effector y (mm)"=w362, "target x (mm)"=w361, "target y (mm)"=w360, "Theta 1"=w353, "Theta 2"=w352, "Omega 1"=w351, "Omega 2"=w350, "timestamp"=w349) -> (w356:T32)
                  n98 = RT FIFO Write(0:w358, 1:w356, 3:w357) -> (8:w355:refnum<k33>, 11:w354:errorcluster)  [unwired: 2 in, 2 out]
                }
              }
              n99 = Bundle By Name(cluster=T26 {"link 2 x (mm)"=0.0, "link 2 y (mm)"=0.0, "link 1 x (mm)"=0.0, "link 1 y (mm)"=0.0} ("current position data"), "link 2 x (mm)"=w168, "link 2 y (mm)"=w167, "link 1 x (mm)"=w187, "link 1 y (mm)"=w186) -> (w190:T26)
              n100 = shared-variable ".\\myPAM.lvlib\\current position data"(w190) -> ()  [unwired: 1 in, 1 out]
              n101 = shared-variable "NI-myRIO-V-Sim\\justindatasavetest.lvlib\\currentx"(w168) -> ()  [unwired: 1 in, 1 out]
              n102 = shared-variable "NI-myRIO-V-Sim\\justindatasavetest.lvlib\\currenty"(w167) -> ()  [unwired: 1 in, 1 out]
              n103 = shared-variable "NI-myRIO-V-Sim\\justindatasavetest.lvlib\\targetx"(w166) -> ()  [unwired: 1 in, 1 out]
              n104 = shared-variable "NI-myRIO-V-Sim\\justindatasavetest.lvlib\\targety"(w165) -> ()  [unwired: 1 in, 1 out]
              n105 = shared-variable "NI-myRIO-V-Sim\\justindatasavetest.lvlib\\timestamp"(w164) -> ()  [unwired: 1 in, 1 out]
              n106 = call "PtByPtFilter.vi"("parameter cluster"=w202, "Mode"=w199, "demand"=w204, "max speed"=w201, "dt"=w197, "error in"=w196, "reset"=w198) -> ("filtered signal"=w203:dbl, "error out"=w194:errorcluster)  [unwired: 7 in]
              n107 = call "PtByPtFilter.vi"("parameter cluster"=w202, "Mode"=w199, "demand"=w206, "max speed"=w201, "dt"=w197, "error in"=w196, "reset"=w198) -> ("filtered signal"=w205:dbl, "error out"=w195:errorcluster)  [unwired: 7 in]
              n108 = To Word Integer(number=w203) -> (16bit integer=w181:i16)
              n109 = Merge Errors(w195, w194) -> (w193:errorcluster)
              n110 = To Word Integer(number=w205) -> (16bit integer=w182:i16)
              n111 = disable-structure shown="Enabled" {
                disable-tunnel: w182 -> [w227 w234]
                disable-tunnel: w181 -> [w226 w233]
                disable-tunnel: [w221 w230] -> w178
                disable-tunnel: [w220 w229] -> w177
                disable-tunnel: [w221 _] -> w180
                disable-tunnel: [w220 _] -> w179
                frame Enabled {
                  w224 = 0.015 ("upper limit")
                  w228 = i16 1000 ("y")
                  n112 = Divide(x=w227, y=w228) -> (x/y=w221:dbl)
                  n113 = Divide(x=w226, y=w228) -> (x/y=w220:dbl)
                  n114 = Greater Than 0?(x=w221) -> (x > 0?=w225:bool)
                  n115 = Negate(x=w224) -> (-x=w223:dbl)
                  n116 = Select(t=w224, s=w225, f=w223) -> (s? t:f=w222:dbl)
                  n117 = Add(x=w222, y=w221) -> ()  [unwired: 1 out]
                }
                frame Disabled {
                  (unwired) u16 10 ("Pulse 1 Wait (ms)")
                  # "Full Rev - 1ms\nStop - 1.5ms\nFull Fwds - 2ms"
                  # "Send Pulse period every 10ms"
                  n118 = Build Array(w234, w233) -> (w232:i16[])
                  n119 = for {
                    tunnel: w232 -> [w238] mode=indexing
                    tunnel: [w239] -> w231 mode=indexing
                    n120 = Add(x=i16 1500 ("y"), y=w238) -> (x+y=w237:i16)
                    n121 = Divide(x=w237, y=1000000.0) -> (x/y=w235:dbl)
                    n122 = Multiply(x=w235, y=40000000.0) -> (x*y=w239:dbl)
                  }
                  n123 = Index Array(array=w231) -> (element #1=w230:dbl, element #2=w229:dbl)  [unwired: 2 in]
                }
              }
              "LINK2_DEMAND" <- w177
              "LINK1_DEMAND" <- w178
              n124 = xnode "Read/Write Control"("FPGA VI Reference In"=w207, "error in"=w193, "Link_1 Duty"=w180, "Link_2 Duty"=w179, "LINK1_DRIVE_ENABLED"=w176, "LINK2_DRIVE_ENABLED"=w176, "Enable Output V"=w176) -> ("FPGA VI Reference Out"=w208:T30, "error out"=w192:errorcluster)
              n125 = shared-variable ".\\myPAM.lvlib\\Operating?"() -> (w219:bool)  [unwired: 1 in, 1 out]
              n126 = node-c288() -> ()  [unwired: 1 in, 1 out]
            }
            n127 = while {
              tunnel: w154 -> [w383]
              tunnel: w148 -> [w382]
              tunnel: [w377] -> w152
              tunnel: [w378] -> w150
              tunnel: w143 -> [w379]
              stop <- w380 stop-if-true
              n128 = RT FIFO Read(0:w383, 2:-1 ("timeout in ms (0)"), 3:w382) -> (8:w377:refnum<k33>, 9:w376:T32, 11:w380:errorcluster)  [unwired: 1 in, 2 out]
              n129 = call "Log Data.vi"("error in"=w380, "data for logging"=w376, "module reference in"=w379) -> ("error out"=w378:errorcluster)  [unwired: 7 in, 1 out]
            }
            n130 = while {
              tunnel: w142 -> [w375]
              tunnel: w148 -> [w374]
              tunnel: [w370] -> w145
              stop <- w371 continue-if-true
              n131 = call "Check for Message.vi"("error in"=w374, "module reference"=w375) -> ("error out"=w372:errorcluster, "new element available"=w373:bool)  [unwired: 8 in]
              n132 = Not(x=w373) -> (.not. x?=w371:bool)
              n133 = shared-variable ".\\myPAM.lvlib\\Operating?"(w371, error in=w372) -> (error out=w370:errorcluster)
            }
            n134 = Not A Number/Path/Refnum?(number/path/refnum=w152) -> (NaN/Path/Refnum?=w151:bool)
            n135 = Select(t=errorcluster {"status"=FALSE, "code"=0, "source"=""}, s=w151, f=w150) -> (s? t:f=w146:errorcluster)
            n136 = node-c288(w162) -> ()  [unwired: 1 out]
            n137 = RT FIFO Delete(0:w156, 3:w155) -> (11:w147:errorcluster)  [unwired: 1 in]
            n138 = Merge Errors(w128, w147, w146, w145) -> (w144:errorcluster)
          }
          frame "shutdown" {
            w384 = FALSE
            w386 = i16 0 ("LINK1_DEMAND_PWM")
            n139 = disable-structure shown="Disabled" {
              frame Disabled {
                w393 = i16 1500  # Stop Pulse Period
                n140 = Divide(x=w393, y=1000000.0) -> (x/y=w395:dbl)
                n141 = Multiply(x=w395, y=40000000.0) -> ()  [unwired: 1 out]
              }
              frame Enabled {
              }
            }
            n142 = xnode "Read/Write Control"("FPGA VI Reference In"=w385, "error in"=w388, "LINK1_DEMAND_PWM"=w386, "LINK2_DEMAND_PWM"=w386, "LINK1_DRIVE_ENABLED"=w384, "LINK2_DRIVE_ENABLED"=w384) -> ("FPGA VI Reference Out"=w387:T30, "error out"=w389:errorcluster)
            n143 = xnode "Close FPGA VI Reference"("FPGA VI Reference In"=w387, "error in"=w389) -> ("error out"=w392:errorcluster)
            n144 = call <vilib>:"Clear Errors.vi"("error in (no error)"=w392) -> ("error out"=w390:errorcluster)  [unwired: 5 in, 1 out]
          }
          frame "disable motors" {
            w397 = FALSE
            w403 = i16 0 ("LINK1_DEMAND_PWM")
            n145 = call "Log Event.vi"("error in"=w401, "event"="Motors Disabled", "module reference in"=w399) -> ("error out"=w400:errorcluster)  [unwired: 7 in, 1 out]
            n146 = disable-structure shown="Disabled" {
              frame Disabled {
                w407 = i16 1500  # Stop Pulse Period
                n147 = Divide(x=w407, y=1000000.0) -> (x/y=w409:dbl)
                n148 = Multiply(x=w409, y=40000000.0) -> ()  [unwired: 1 out]
              }
              frame Enabled {
              }
            }
            n149 = xnode "Read/Write Control"("FPGA VI Reference In"=w404, "error in"=w400, "LINK1_DEMAND_PWM"=w403, "LINK2_DEMAND_PWM"=w403, "LINK1_DRIVE_ENABLED"=w397, "LINK2_DRIVE_ENABLED"=w397) -> ("FPGA VI Reference Out"=w402:T30, "error out"=w405:errorcluster)
          }
        }
      }
    }
    n150 = call "Handle Error.vi"("module reference in"=w28, "error in"=w30) -> ("error out"=w29:errorcluster)  [unwired: 9 in]
  }
  n151 = while {
    tunnel: w22 -> [w416]
    tunnel: [w415] -> w21
    tunnel: w3 -> [w413]
    tunnel: [w412] -> w15
    tunnel: w13 -> [w411]
    stop <- w414 stop-if-true
    # "Shutdown user event listener"
    n152 = case shown="No Error" w413 {
      selector: w413 -> [w419 _]
      tunnel: w416 -> [w422 w431]
      tunnel: [w421 w431] -> w415
      tunnel: [w420 TRUE] -> w414
      tunnel: [w418 errorcluster {"status"=FALSE, "code"=0, "source"=""} ("error out")] -> w412
      tunnel: w411 -> [w417 _]
      frame No Error {
        n153 = event shown="[1] <shutdown user event>: User Event" {
          selector: w422 -> [_ _]
          dyn-events: [_ _] -> w421
          timeout: _ -> [_ _]
          tunnel: w419 -> [w423 w427]
          tunnel: [w423 w426] -> w418
          tunnel: [_ TRUE] -> w420
          tunnel: w417 -> [_ w425]
          event Timeout {
            n154 = event-data() -> ()  [unwired: 1 in, 3 out]
          }
          event User Event {
            n155 = event-data() -> ()  [unwired: 1 in, 1 out]
            n156 = call "Enqueue Message.vi"("high priority"=TRUE, "message"=Messages."shutdown", "error in"=w427, "module reference in"=w425) -> ("error out"=w426:errorcluster)  [unwired: 6 in, 1 out]
          }
        }
      }
      frame Error {
      }
    }
  }
  n157 = Unregister For Events(event registration refnum=w21, error in=w15) -> (error out=w16:errorcluster)
  n158 = Merge Errors(w20, w16) -> (→"error out":errorcluster)
